vi "Multiply Gains.vi"(1 "Other Gain":dbl[](array[numeric]), 2 "Gain":dbl[](array[numeric])) -> (0 "Gain x Other Gain":dbl[](array[numeric]))   [LabVIEW 2016]
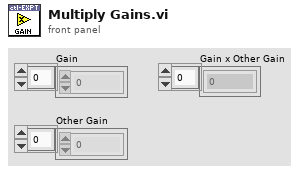
[diagram p1: front panel]
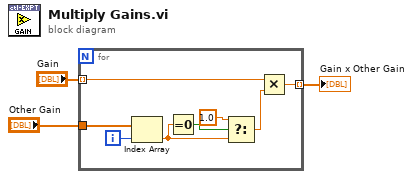
[diagram p0: block diagram]
diagram:
  n1 = for {
    tunnel: "Gain" -> [w11] mode=indexing
    tunnel: "Other Gain" -> [w9]
    tunnel: [w10] -> w3 mode=indexing
    i -> [w8]
    n2 = Index Array(array=w9, index=w8) -> (element=w5:dbl)
    n3 = Equal To 0?(x=w5) -> (x = 0?=w7:bool)
    n4 = Select(t=1.0, s=w7, f=w5) -> (s? t:f=w6:dbl)
    n5 = Multiply(x=w11, y=w6) -> (x*y=w10:dbl)
  }
  "Gain x Other Gain" <- w3
